vi "Slope_Calculator (SubVI).vi"(6 "X1":dbl, 9 "X2":dbl, 10 "Y1":dbl, 11 "Y2":dbl) -> (3 "Numeric":dbl)   [LabVIEW 2020]
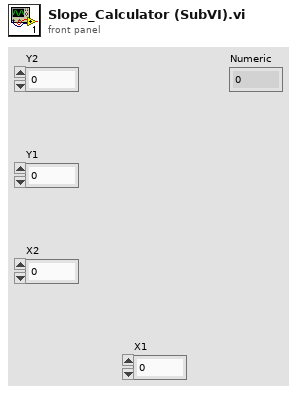
[diagram p1: front panel]
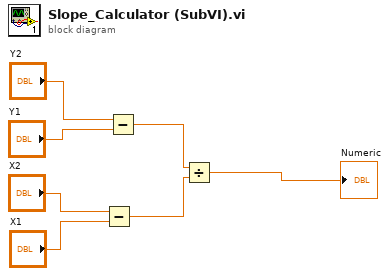
[diagram p0: block diagram]
diagram:
  n1 = Subtract(x="X2", y="X1") -> (x-y=w6:dbl)
  n2 = Subtract(x="Y2", y="Y1") -> (x-y=w5:dbl)
  n3 = Divide(x=w5, y=w6) -> (x/y=→"Numeric":dbl)
